vi "triatge_dadesFinal_linia.vi"(8 "ShiftReg LEFT":T3, 11 "String in":string) -> (0 "ShiftReg RIGHT":T2, 3 "DADES":T1)   [LabVIEW 2018]
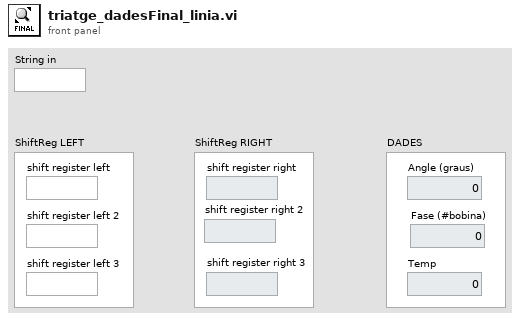
[diagram p1: front panel]
types:
  T1 = cluster{"Angle (graus)":dbl, "Fase (#bobina)":dbl, "Temp":dbl}
  T2 = cluster{"shift register right":string, "shift register right 2":string, "shift register right 3":string}
  T3 = cluster{"shift register left":string, "shift register left 2":string, "shift register left 3":string}
  T4 = cluster{"Data Out":dbl, "Data Out":dbl, "Data Out":dbl}
  T5 = cluster{"shift register right":string, "shift register right":string, "shift register right":string}
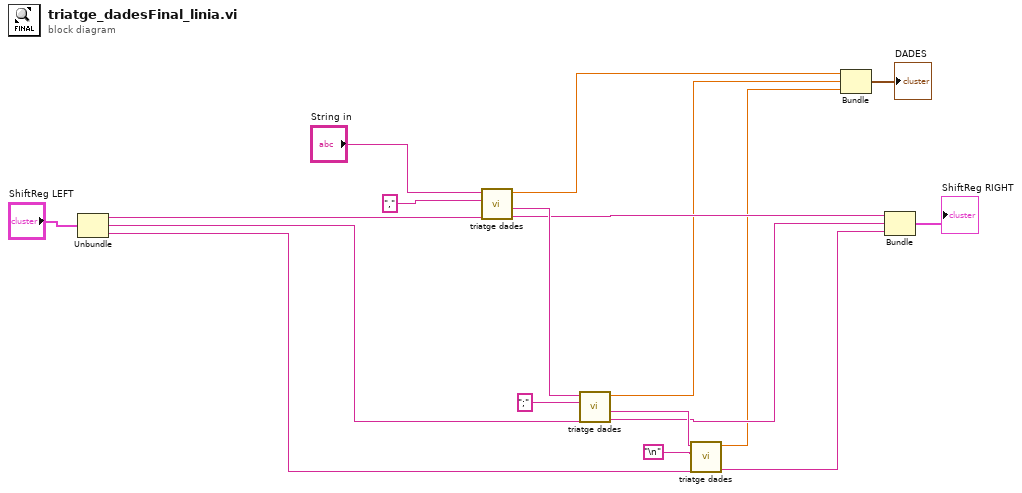
[diagram p0: block diagram]
diagram:
  n1 = Unbundle("ShiftReg LEFT") -> ("shift register left"=w7:string, "shift register left 2"=w6:string, "shift register left 3"=w5:string)
  n2 = call "triatge dades.vi"("shift register left"=w7, "dada a buscar"=",", "String in"="String in") -> ("shift register right"=w11:string, "String Out"=w17:string, "Data Out"=w3:dbl)  [unwired: 5 in, 1 out]
  n3 = call "triatge dades.vi"("shift register left"=w6, "dada a buscar"=";", "String in"=w17) -> ("shift register right"=w10:string, "String Out"=w14:string, "Data Out"=w2:dbl)  [unwired: 5 in, 1 out]
  n4 = call "triatge dades.vi"("shift register left"=w5, "dada a buscar"="\n", "String in"=w14) -> ("shift register right"=w9:string, "Data Out"=w1:dbl)  [unwired: 5 in, 2 out]
  n5 = Bundle("Data Out"=w3, "Data Out"=w2, "Data Out"=w1) -> (→"DADES":T4)  [unwired: 1 in]
  n6 = Bundle("shift register right"=w11, "shift register right"=w10, "shift register right"=w9) -> (→"ShiftReg RIGHT":T5)  [unwired: 1 in]
